vi "Init Runtime.vi"(8 "error in (no error)":errorcluster, 10 "data allocations":T1, 11 "Update Tag Config in":refnum<class "Update Tag Config.lvclass">) -> (0 "error out":errorcluster, 2 "Skip":bool, 3 "Update Tag Config out":refnum<class "Update Tag Config.lvclass">)   [LabVIEW 2015, in "Update Tag Config.lvclass"]
uses:
  Update Tag Config.lvclass
  <vilib>/NI/Tag Bus Module Framework/channel/data tables.ctl
  <vilib>/NI/Tag Bus/dictionary/data dictionary.lvclass
  <vilib>/NI/Tag Bus/dictionary table pair.ctl
  <vilib>/NI/Tag Bus/table/data table.ctl
  Update Tag Step/Update Tag.lvclass
  <vilib>/NI/Tag Bus Module Framework/channel/TBM channel.lvclass/TBM channel.ctl
  <vilib>/NI/Tag Bus/tag/tag descriptor.lvclass/tag descriptor.ctl
  <vilib>/NI/Tag Bus/dictionary/locate tag.vi
  <vilib>/NI/Tag Bus Module Framework/channel/TBM channel.lvclass
  <vilib>/NI/Tag Bus/tag/tag descriptor.lvclass
  <vilib>/NI/Tag Bus/table/data table.lvlib
  <vilib>/NI/Tag Bus/tag bus.lvlib
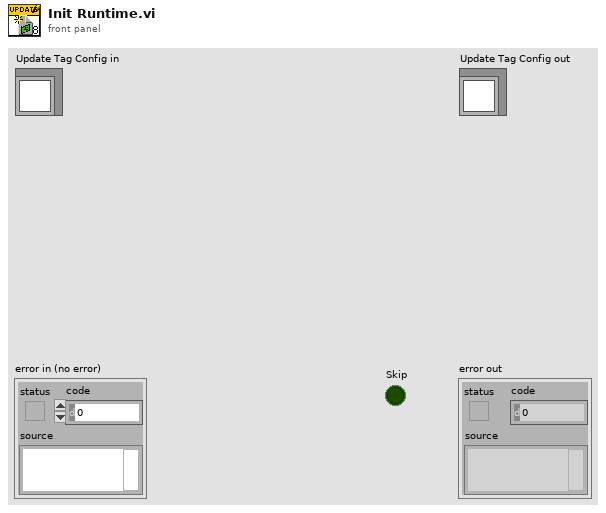
[diagram p1: front panel]
types:
  T1 = typedef "TBM channel.lvclass/data tables.ctl" = cluster{"input data":T2, "processing parameter":T2, "processing result":T2, "output data":T2}
  T2 = typedef "tag bus.lvlib/dictionary table pair.ctl" = cluster{"data dictionary":refnum<class "data dictionary.lvclass">, "data table":T3}
  T3 = typedef "tag bus.lvlib/data table.lvlib/data table.ctl" = cluster{"Double":dbl[], "Single":sgl[], "I64":i64[], "I32":i32[], "I16":i16[], "I8":i8[], "U64":u64[], "U32":u32[], "U16":u16[], "U8":u8[], "Boolean":bool[], "String":string[], "Array of Double":cluster{"DBL Array":dbl[]}[], "Array of Single":cluster{"SGL Array":sgl[]}[], "Array of I64":cluster{"I64 Array":i64[]}[], "Array of I32":cluster{"I32 Array":i32[]}[], "Array of I16":cluster{"I16 Array":i16[]}[], "Array of I8":cluster{"I8 Array":i8[]}[], "Array of U64":cluster{"U64 Array":u64[]}[], "Array of U32":cluster{"U32 Array":u32[]}[], "Array of U16":cluster{"U16 Array":u16[]}[], "Array of U8":cluster{"U8 Array":u8[]}[], "Array of Boolean":cluster{"Boolean Array":bool[]}[], "Array of String":cluster{"String Array":string[]}[]}
  T4 = typedef "tag bus.lvlib/tag descriptor.lvclass/Data Type.ctl" = enum16{"Double", "Single", "I64", "I32", "I16", "I8", "U64", "U32", "U16", "U8", "Boolean", "String", "Array of Double", "Array of Single", "Array of I64", "Array of I32", "Array of I16", "Array of I8", "Array of U64", "Array of U32", "Array of U16", "Array of U8", "Array of Boolean", "Array of String"}
  T5 = typedef "TBM channel.lvclass/channel classification.ctl" = enum16{"input data", "output data", "processing parameter", "processing result"}
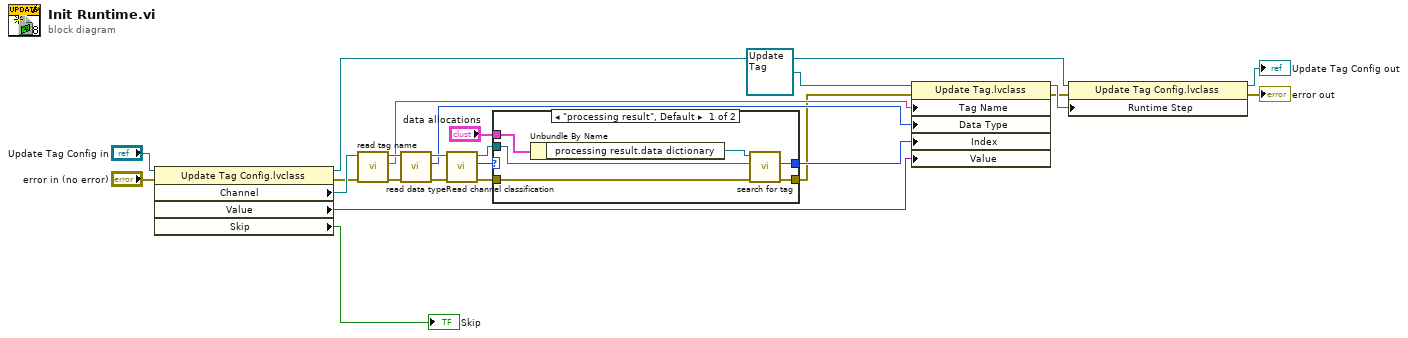
[diagram p0: block diagram]
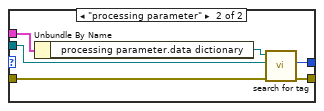
[diagram p2: hidden frame]
diagram:
  n1 = property class="Update Tag Config.lvclass"(reference="Update Tag Config in", error in="error in (no error)") -> (reference out=w23:refnum<class "Update Tag Config.lvclass">, error out=w8:errorcluster, "Channel"=w17:refnum<class "TBM channel.lvclass">, "Value"=w2:variant, "Skip"=→"Skip":bool)
  n2 = call <vilib>:"read tag name.vi"("error in"=w8, "system tag in"=w17) -> ("error out"=w7:errorcluster, "name"=w14:string, "system tag out"=w16:refnum<class "TBM channel.lvclass">)  [unwired: 7 in]
  n3 = call <vilib>:"read data type.vi"("error in"=w7, "system tag in"=w16) -> ("error out"=w6:errorcluster, "data type"=w13:T4, "system tag out"=w15:refnum<class "TBM channel.lvclass">)  [unwired: 7 in]
  n4 = call <vilib>:"Read channel classification.vi"("error in"=w6, "channel in"=w15) -> ("error out"=w5:errorcluster, "channel classification"=w12:T5, "channel out"=w10:refnum<class "TBM channel.lvclass">)  [unwired: 7 in]
  n5 = case shown="\"processing result\", Default" w12 {
    tunnel: "data allocations" -> [w29 w36]
    tunnel: w10 -> [w25 w34]
    tunnel: [w28 w33] -> w9
    tunnel: w5 -> [w27 w32]
    tunnel: [w26 w31] -> w4
    frame "processing result", Default {
      n6 = Unbundle By Name(w29) -> ("processing result.data dictionary"=w30:refnum<class "data dictionary.lvclass">)
      n7 = call <vilib>:"search for tag.vi"("error in"=w27, "system tag"=w25, "data dictionary in"=w30) -> ("error out"=w26:errorcluster, "index"=w28:i32)  [unwired: 6 in, 1 out]
    }
    frame "processing parameter" {
      n8 = Unbundle By Name(w36) -> ("processing parameter.data dictionary"=w35:refnum<class "data dictionary.lvclass">)
      n9 = call <vilib>:"search for tag.vi"("error in"=w32, "system tag"=w34, "data dictionary in"=w35) -> ("error out"=w31:errorcluster, "index"=w33:i32)  [unwired: 6 in, 1 out]
    }
  }
  n10 = property class="Update Tag.lvclass"(reference=refnum<class "Update Tag.lvclass"> refnum ("Update Tag.lvclass"), error in=w4, "Tag Name"=w14, "Data Type"=w13, "Index"=w9, "Value"=w2) -> (reference out=w21:refnum<class "Update Tag.lvclass">, error out=w20:errorcluster)
  n11 = property class="Update Tag Config.lvclass"(reference=w23, error in=w20, "Runtime Step"=w21) -> (reference out=→"Update Tag Config out":refnum<class "Update Tag Config.lvclass">, error out=→"error out":errorcluster)
